vi "Set Variant.vi"(8 "error in (no error)":errorcluster, 10 "Variant":variant, 11 "Type Serializer in":refnum<class "Basic Type.lvclass">) -> (0 "error out":errorcluster, 3 "Type Serializer out":refnum<class "Basic Type.lvclass">)   [LabVIEW 2020, in "Protobuf RAW.lvlib" / "Basic Type.lvclass"]
uses:
  Tag/Basic Type.lvclass
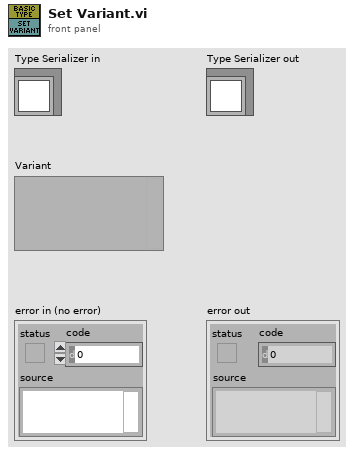
[diagram p1: front panel]
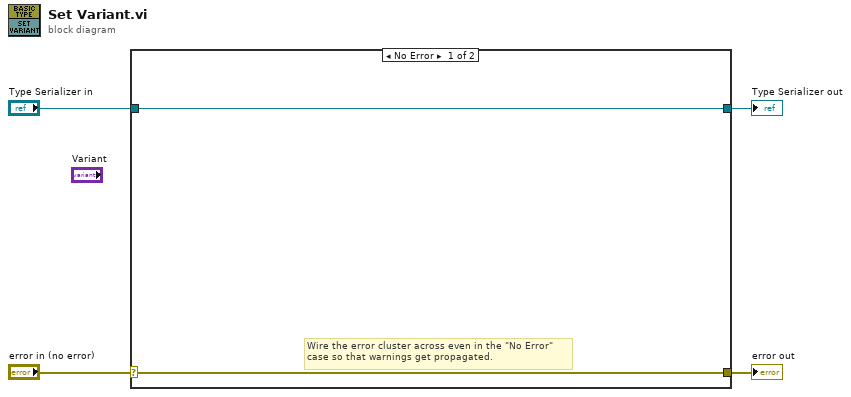
[diagram p0: block diagram]
diagram:
  n1 = case shown="No Error" "error in (no error)" {
    selector: "error in (no error)" -> [w5 w8]
    tunnel: [w5 w8] -> w3
    tunnel: [w6 w7] -> w1
    tunnel: "Type Serializer in" -> [w6 w7]
    frame No Error {
      # "Wire the error cluster across even in the \"No Error\"\ncase so that warnings get propagated."
    }
    frame Error {
    }
  }
  "error out" <- w3
  "Type Serializer out" <- w1
